vi "subGeneratePackets.vi"(4 "DTMF Settings":T1={"Phone Number"="", "Dial Tone"=FALSE, "Quantization Level"=4, "\nGray Encoding"=FALSE} {"Quantization Level" items=["2"=2, "4"=4, "8"=8, "16"=16]}, 5 "PSK system parameters":T3, 6 "Packet Parameters":T2, 7 "Packet Pad \n[samples]":i32, 8 "PN sequence order\nfor Sync Bits":i32, 9 "Pulse Shaping Filter Parameters":T4, 10 "Tx IQ Sampling\nRate [s/sec]":dbl, 11 "Samples per Symbol":i32) -> (0 "TX DTMF Signal":dbl[][](array[numeric]), 1 "Symbol Rate":dbl, 2 "Packets":cluster{"t0":dbl, "dt":dbl, "Y":cdb[]}[](array[cluster]), 3 "Number of Packets":i32)   [LabVIEW 2011]
panel:
  in  "size(s)":i32
  out "File Length (bits)":i32
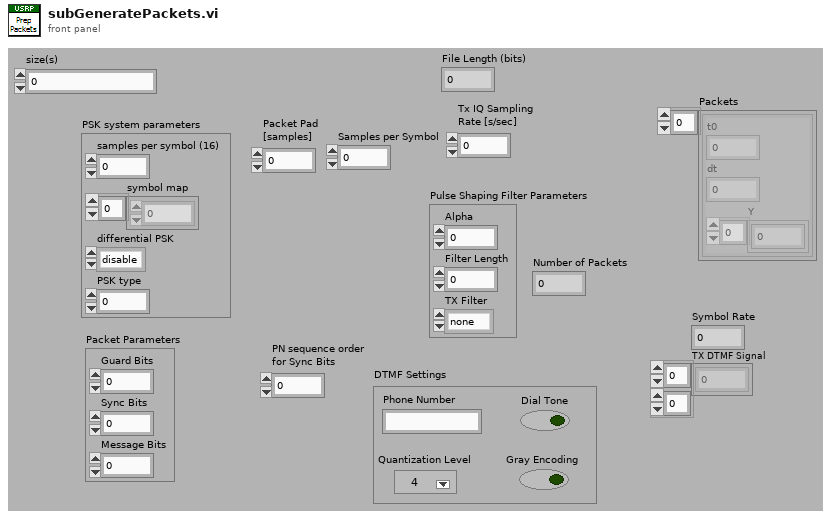
[diagram p1: front panel]
types:
  T1 = cluster{"Phone Number":string, "Dial Tone":bool, "Quantization Level":u16, "\nGray Encoding":bool}
  T2 = cluster{"Guard Bits ":i32, "Sync Bits":i32, "Message Bits":i32}
  T3 = cluster{"samples per symbol (16)":i32, "symbol map":cdb[], "differential PSK":enum16{"disable", "enable"}, "PSK type":u16}
  T4 = cluster{"Alpha":dbl, "Filter Length":i32, "TX Filter":enum16{"none", "Raised Cosine", "Root Raised Cos", "Gaussian"}}
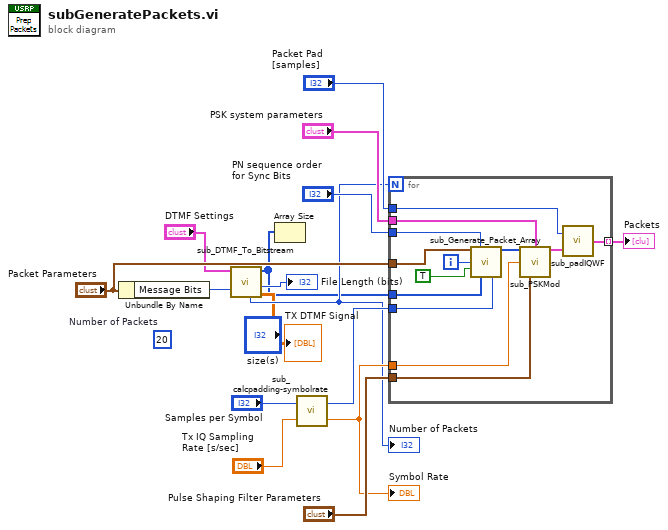
[diagram p0: block diagram]
diagram:
  (unwired) 20  # Number of Packets
  n1 = Unbundle By Name("Packet Parameters") -> ("Message Bits"=w6:i32)
  n2 = call "sub_DTMF_To_Bitstream.vi"("Packet\nMessage Length (bits)"=w6, "DTMF Settings"="DTMF Settings") -> ("TX DTMF Signal"=→"TX DTMF Signal":dbl[][], "File Length (bits)"=→"File Length (bits)":i32, "message bitstream"=w1:i8[], "Number of Packets"=w5:i32)  [unwired: 6 in]
  "Number of Packets" <- w5
  n3 = Array Size(array=w1) -> ()  [unwired: 1 out]
  n4 = call "sub_calcpadding-symbolrate.vi"("Tx IQ Sampling\nRate [s/sec]"="Tx IQ Sampling\nRate [s/sec]", "Samples per Symbol"="Samples per Symbol") -> ("Symbol Rate"=w8:dbl, "Padding Bits"=w10:i32)
  "Symbol Rate" <- w8
  n5 = for {
    N: w5 -> [_]
    tunnel: "Packet Parameters" -> [w27]
    tunnel: [w20] -> w12 mode=indexing
    tunnel: w1 -> [w28]
    tunnel: "PN sequence order\nfor Sync Bits" -> [w26]
    tunnel: w10 -> [w25]
    tunnel: "PSK system parameters" -> [w23]
    tunnel: w8 -> [w22]
    tunnel: "Pulse Shaping Filter Parameters" -> [w21]
    tunnel: "Packet Pad \n[samples]" -> [w18]
    i -> [w29]
    n6 = call "sub_Generate_Packet_Array.vi"("Packet Parameters"=w27, "PN sequence order\nfor Sync"=w26, "Packet Number"=w29, "User defined bitstream?"=TRUE ("Message Type"), "user  bitstream"=w28, "Cyclic Padding Bits"=w25) -> ("Output Packet"=w24:i8[])  [unwired: 9 in]
    n7 = call "sub_PSKMod.vi"("Packet to Transmit"=w24, "PSK system parameters"=w23, "Symbol Rate, Hz"=w22, "filter parameters"=w21) -> ("output complex waveform"=w19:cluster{"t0":dbl, "dt":dbl, "Y":cdb[]})  [unwired: 9 in, 2 out]
    n8 = call "sub_padIQWF.vi"("input complex waveform"=w19, "Packet Pad \n[samples]"=w18) -> ("output complex waveform"=w20:cluster{"t0":dbl, "dt":dbl, "Y":cdb[]})
  }
  "Packets" <- w12
